vi "Temp Aleatoria.vi"(10 "Limite Minimo":dbl, 11 "Limite Maximo":dbl) -> (3 "Numeric":dbl)   [LabVIEW 2020]
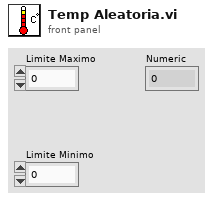
[diagram p1: front panel]
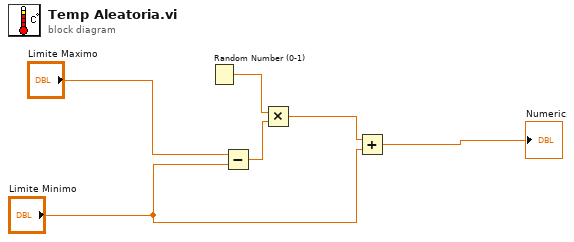
[diagram p0: block diagram]
diagram:
  n1 = Random Number (0-1)() -> (number: 0 to 1=w3:dbl)
  n2 = Subtract(x="Limite Maximo", y="Limite Minimo") -> (x-y=w2:dbl)
  n3 = Multiply(x=w3, y=w2) -> (x*y=w5:dbl)
  n4 = Add(x=w5, y="Limite Minimo") -> (x+y=→"Numeric":dbl)
